vi "Cmd.ClearError.vi"(6 "Timeout [ms] (1000)":i32=1000, 8 "error in":errorcluster, 11 "cID in":refnum<k5>) -> (0 "error out":errorcluster, 3 "cID out":refnum<k5>)   [LabVIEW 2016]
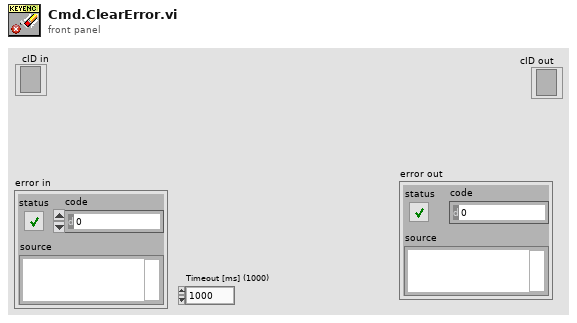
[diagram p1: front panel]
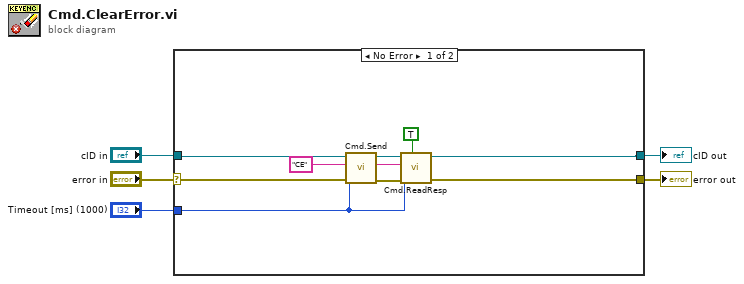
[diagram p0: block diagram]
diagram:
  n1 = case shown="No Error" "error in" {
    selector: "error in" -> [w13 w15]
    tunnel: "Timeout [ms] (1000)" -> [w10 _]
    tunnel: "cID in" -> [w14 w16]
    tunnel: [w9 w16] -> w2
    tunnel: [w8 w15] -> w1
    frame No Error {
      w7 = "CE"
      n2 = call "Cmd.Send.vi"("error in (no error)"=w13, "Timeout [ms] (1000)"=w10, "Command"=w7, "connection ID"=w14) -> ("error out"=w11:errorcluster, "connection ID out"=w12:refnum<k5>)  [unwired: 6 in]
      n3 = call "Cmd.ReadResp.vi"("IgnoreError"=TRUE, "error in (no error)"=w11, "Timeout [ms] (1000)"=w10, "Request"=w7, "connection ID"=w12) -> ("error out"=w8:errorcluster, "connection ID out"=w9:refnum<k5>)  [unwired: 4 in, 1 out]
    }
    frame Error {
    }
  }
  "cID out" <- w2
  "error out" <- w1
